vi "33 累加到66.vi"() -> ()   [LabVIEW 2023]
panel:
  out "33 累加到 66":i32
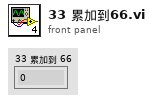
[diagram p1: front panel]
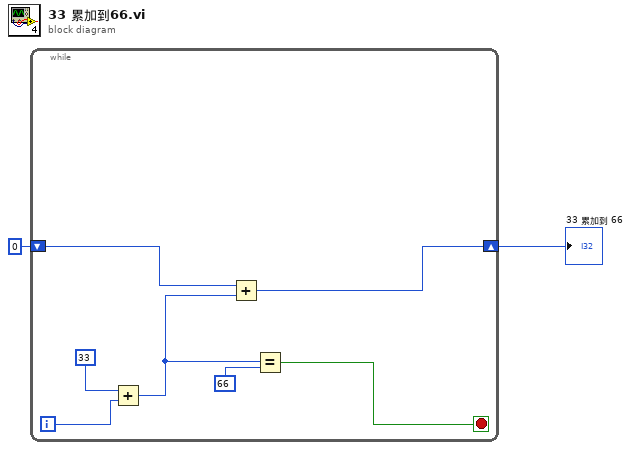
[diagram p0: block diagram]
diagram:
  n1 = while {
    shift-right: [w7] -> w1
    shift-left: 0 -> [w6]
    i -> [w9]
    stop <- w3 stop-if-true
    n2 = Add(x=33, y=w9) -> (x+y=w5:i32)
    n3 = Add(x=w6, y=w5) -> (x+y=w7:i32)
    n4 = Equal?(x=w5, y=66) -> (x = y?=w3:bool)
  }
  "33 累加到 66" <- w1
